vi "Intake_Teleop.vi"(11 "Joystick_In":T1) -> ()   [LabVIEW 2019]
uses:
  Utility_VIs/Joystick_Controls.ctl
  Intake_Cluster.ctl
  Intake_States.ctl
  Intake_Globals.vi
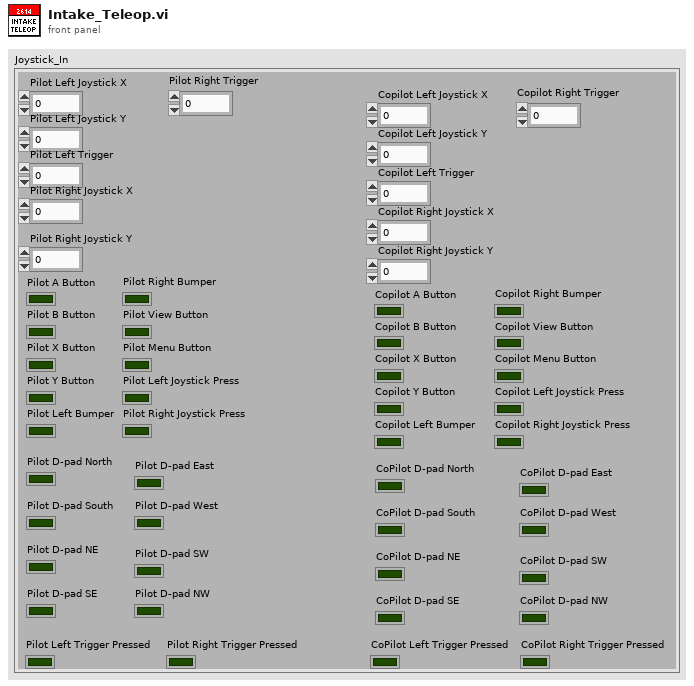
[diagram p1: front panel]
types:
  T1 = typedef "Joystick_Controls.ctl" = cluster{"Pilot Left Joystick X":dbl, "Pilot Left Joystick Y":dbl, "Pilot A Button":bool, "Pilot B Button":bool, "Pilot X Button":bool, "Pilot Y Button":bool, "Pilot Left Bumper":bool, "Pilot Right Bumper":bool, "Pilot View Button":bool, "Pilot Menu Button":bool, "Pilot Left Joystick Press":bool, "Pilot Right Joystick Press":bool, "Pilot Left Trigger":dbl, "Pilot Right Joystick X":dbl, "Pilot Right Joystick Y":dbl, "Pilot Right Trigger":dbl, "Copilot Left Joystick X":dbl, "Copilot Left Joystick Y":dbl, "Copilot A Button":bool, "Copilot B Button":bool, "Copilot X Button":bool, "Copilot Y Button":bool, "Copilot Left Bumper":bool, "Copilot Right Bumper":bool, "Copilot View Button":bool, "Copilot Menu Button":bool, "Copilot Left Joystick Press":bool, "Copilot Right Joystick Press":bool, "Copilot Left Trigger":dbl, "Copilot Right Joystick X":dbl, "Copilot Right Joystick Y":dbl, "Copilot Right Trigger":dbl, "Pilot D-pad North":bool, "Pilot D-pad South":bool, "Pilot D-pad East":bool, "Pilot D-pad West":bool, "Pilot D-pad NE ":bool, "Pilot D-pad SE":bool, "Pilot D-pad SW":bool, "Pilot D-pad NW":bool, "CoPilot D-pad North":bool, "CoPilot D-pad South":bool, "CoPilot D-pad East":bool, "CoPilot D-pad West":bool, "CoPilot D-pad NE":bool, "CoPilot D-pad SE":bool, "CoPilot D-pad SW":bool, "CoPilot D-pad NW":bool, "Pilot Left Trigger Pressed":bool, "Pilot Right Trigger Pressed":bool, "CoPilot Left Trigger Pressed":bool, "CoPilot Right Trigger Pressed":bool}
  T2 = typedef "Intake_Cluster.ctl" = cluster{"Control_State":T3, "Intake_On":bool, "Intake_Extended":bool, "Intake_Throttle":dbl, "Auto_Notifier":refnum<notifier>, "Parameter_1":dbl, "Parameter_2":dbl, "Step":dbl, "Outtake":bool}
  T3 = typedef "Intake_States.ctl" = enum16{"Manual_Control", "Compliant_Intake", "Command_RunIntake"}
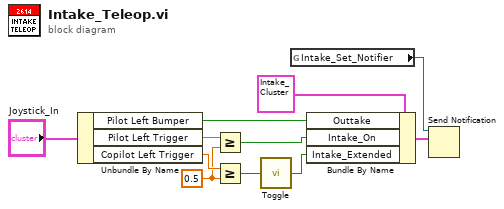
[diagram p0: block diagram]
diagram:
  w1 = 0.5 ("y")
  n1 = Unbundle By Name("Joystick_In") -> ("Pilot Left Bumper"=w4:bool, "Pilot Left Trigger"=w7:dbl, "Copilot Left Trigger"=w2:dbl)
  n2 = Greater Or Equal?(x=w7, y=w1) -> (x >= y?=w6:bool)
  n3 = Greater Or Equal?(x=w2, y=w1) -> (x >= y?=w3:bool)
  n4 = call "Toggle.vi"("Boolean"=w3) -> ("Boolean Out"=w5:bool)
  n5 = global read "Intake_Globals.vi" "Intake_Set_Notifier"() -> (w10:refnum<notifier>)
  n6 = Bundle By Name(cluster=T2 {"Control_State"=enum."Manual_Control", "Intake_On"=FALSE, "Intake_Extended"=FALSE, "Intake_Throttle"=0.0, "Auto_Notifier"=refnum, "Parameter_1"=0.0, "Parameter_2"=0.0, "Step"=0.0, "Outtake"=FALSE} ("notification"), "Outtake"=w4, "Intake_On"=w6, "Intake_Extended"=w5) -> (w8:T2)
  n7 = Send Notification(notification=w8, notifier=w10) -> ()  [unwired: 1 in, 2 out]
